vi "deeplabv3_generate_color_masks.vi"() -> (3 "colors":u32[](array[numeric]))   [LabVIEW 2018]
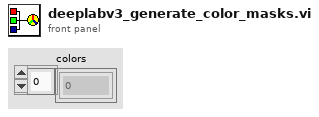
[diagram p1: front panel]
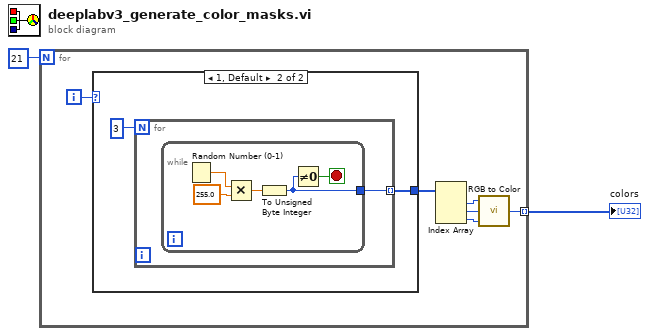
[diagram p0: block diagram]
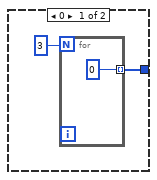
[diagram p2: hidden frame]
diagram:
  n1 = for {
    N: 21 -> [_]
    tunnel: [w3] -> w2 mode=indexing
    i -> [w8]
    n2 = case shown="1, Default" w8 {
      tunnel: [w9 w12] -> w7
      frame 0 {
        n3 = for {
          N: 3 -> [_]
          tunnel: [u8 0] -> w9 mode=indexing
        }
      }
      frame 1, Default {
        n4 = for {
          N: 3 -> [_]
          tunnel: [w14] -> w12 mode=indexing
          n5 = while {
            tunnel: [w15] -> w14
            stop <- w16 stop-if-true
            n6 = Random Number (0-1)() -> (number: 0 to 1=w19:dbl)
            n7 = Multiply(x=w19, y=255.0) -> (x*y=w17:dbl)
            n8 = To Unsigned Byte Integer(number=w17) -> (unsigned 8bit integer=w15:u8)
            n9 = Not Equal To 0?(x=w15) -> (x != 0?=w16:bool)
          }
        }
      }
    }
    n10 = Index Array(array=w7) -> (element #1=w5:u8, element #2=w6:u8, element #3=w4:u8)  [unwired: 3 in]
    n11 = call <vilib>:"RGB to Color.vi"("B"=w4, "G"=w6, "R"=w5) -> ("Color"=w3:u32)
  }
  "colors" <- w2
